vi "Excute.vi"(8 "error in (no error)":errorcluster, 11 "ConcreateComponent in":refnum<class "ConcreateComponent.lvclass">) -> (0 "error out":errorcluster, 3 "ConcreateComponent out":refnum<class "ConcreateComponent.lvclass">)   [LabVIEW 2014, in "ConcreateComponent.lvclass"]
uses:
  ConcreateComponent.lvclass
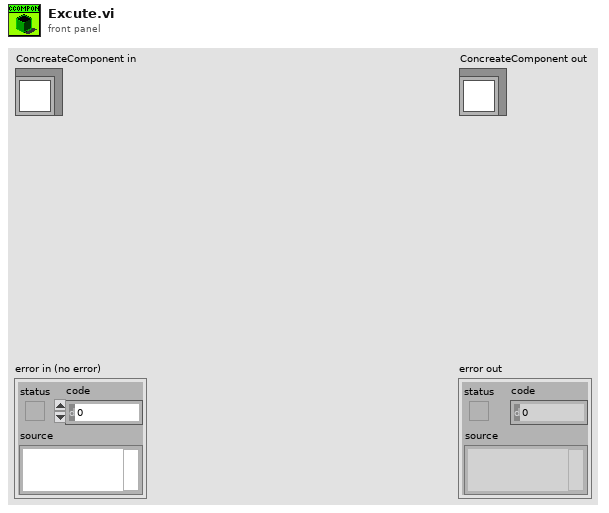
[diagram p1: front panel]
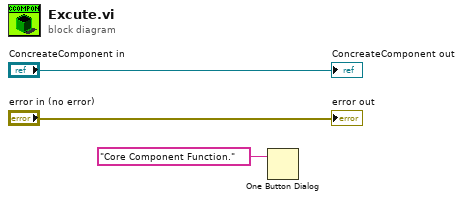
[diagram p0: block diagram]
diagram:
  n1 = One Button Dialog(message="Core Component Function.") -> ()  [unwired: 1 in, 1 out]
  "error out" <- "error in (no error)"
  "ConcreateComponent out" <- "ConcreateComponent in"
